vi "ReadAvailableRecords_5782.vi"(11 "scope params":T1) -> (0 "last record size":u32, 1 "#elements":u32, 2 "record available":bool, 3 "scope params out":T1)   [LabVIEW 2013]
uses:
  controls/scope_params_5782.ctl
  Utilities/Ticker/Ticker.lvclass
  Scope/controls/ScopeMode.ctl
  Config/FPGAref_5782.ctl
  FPGA/DataMode.ctl
  controls/5782_trigger_type.ctl
  <vilib>/rvi/interface/common/niFpgaWaitOnOcc.vi
  <vilib>/Utility/error.llb/Error Cluster From Error Code.vi
  <vilib>/rvi/errors/niLvFpgaAdjustHostInterfaceError.vi
  <vilib>/rvi/interface/nirviMethod/nirviMethod.xnode
  <vilib>/FPGAPlugInAG/Dynamic/niLvFpga_ReadFifo_Dynamic.vi
  <vilib>/rvi/errors/niLvFpgaMergeErrorWithErrorCode.vi
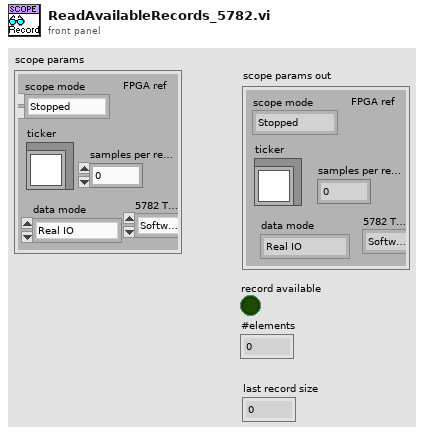
[diagram p1: front panel]
types:
  T1 = typedef "scope_params_5782.ctl" = cluster{"scope mode":T2, "ticker":refnum<class "Ticker.lvclass">, "samples per record":i32, "FPGA ref":T3, "data mode":T4, "5782 Trigger":T5}
  T2 = typedef "ScopeMode.ctl" = enum16{"Stopped", "Single", "Running", "Continuous"}
  T3 = typedef "FPGAref_5782.ctl" = refnum<k20>
  T4 = typedef "DataMode.ctl" = enum16{"Real IO", "Simulated"}
  T5 = typedef "5782_trigger_type.ctl" = enum16{"Software", "Trigger input"}
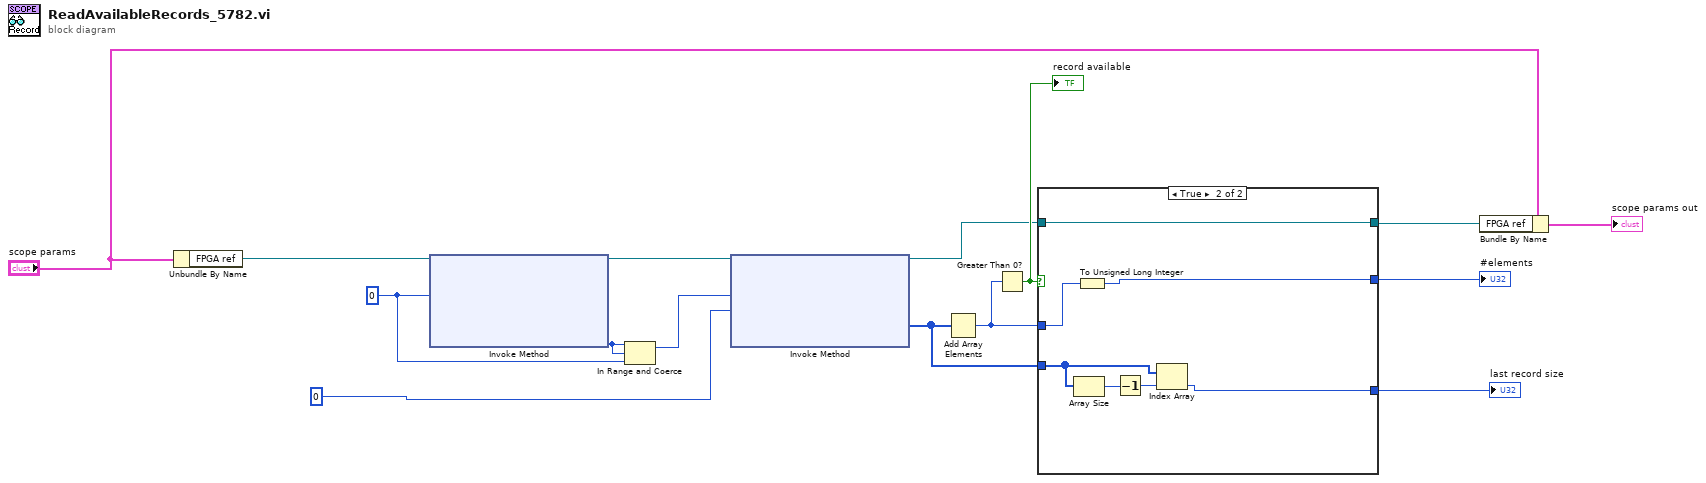
[diagram p0: block diagram]
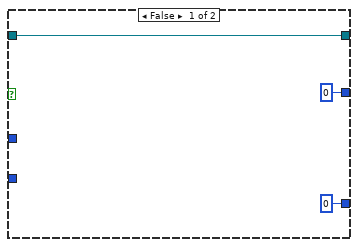
[diagram p2: hidden frame]
diagram:
  w6 = u32 0 ("Number of Elements")
  n1 = Unbundle By Name("scope params") -> ("FPGA ref"=w9:T3)
  n2 = xnode "Invoke Method"("FPGA VI Reference In"=w9, "Number of Elements"=w6) -> ("FPGA VI Reference Out"=w15:T3, "Elements Remaining"=w5:u32)  [unwired: 2 in, 2 out]
  n3 = In Range and Coerce(upper limit=w5, x=w5, lower limit=w6) -> (coerced(x)=w7:u32)  [unwired: 1 out]
  n4 = xnode "Invoke Method"("FPGA VI Reference In"=w15, "Number of Elements"=w7, "Timeout (ms)"=0) -> ("FPGA VI Reference Out"=w4:T3, "Data"=w13:u16[])  [unwired: 1 in, 2 out]
  n5 = Add Array Elements(numeric array=w13) -> (sum=w14:u16)
  n6 = Greater Than 0?(x=w14) -> (x > 0?=w12:bool)
  "record available" <- w12
  n7 = case shown="True" w12 {
    tunnel: w4 -> [w18 w21]
    tunnel: w14 -> [_ w22]
    tunnel: w13 -> [_ w25]
    tunnel: [w18 w21] -> w1
    tunnel: [u32 0 w19] -> w3
    tunnel: [u32 0 w20] -> w2
    frame False {
    }
    frame True {
      n8 = Array Size(array=w25) -> (size(s)=w24:i32)
      n9 = To Unsigned Long Integer(number=w22) -> (unsigned 32bit integer=w20:u32)
      n10 = Decrement(x=w24) -> (x-1=w23:i32)
      n11 = Index Array(array=w25, index=w23) -> (element=w19:u16)
    }
  }
  "last record size" <- w3
  "#elements" <- w2
  n12 = Bundle By Name(cluster="scope params", "FPGA ref"=w1) -> (→"scope params out":T1)
